vi "Destroy.vi"(8 "Error In":errorcluster, 11 "reference in":refnum<class "DinnerMenuEnum.lvclass">) -> (0 "Error Out":errorcluster, 3 "reference out":refnum<class "DinnerMenuEnum.lvclass">)   [LabVIEW 2020, in "DinnerMenuEnum.lvclass"]
uses:
  DinnerMenuEnum.lvclass
  DinnerMenuEnum.lvclass/DinnerMenuEnum.ctl
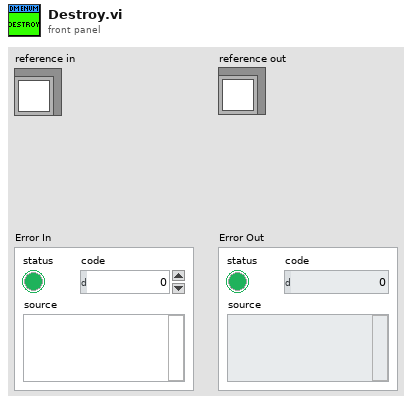
[diagram p1: front panel]
types:
  T1 = typedef "DinnerMenuEnum.lvclass/ObjectAttributes.ctl" = cluster{"_items":refnum<class "Menu.lvclass">[], "_position":i32, "IEnumerator.Current":refnum<class>, "Current":refnum<class "Menu.lvclass">}
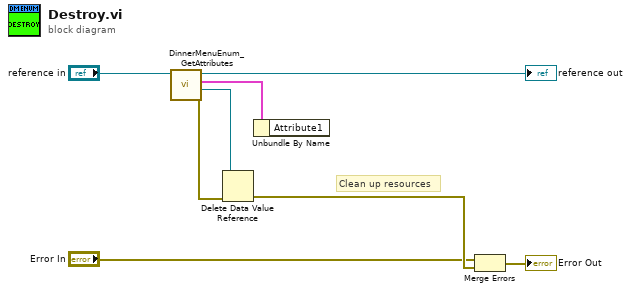
[diagram p0: block diagram]
diagram:
  # "Clean up resources"
  n1 = call "DinnerMenuEnum_GetAttributes.vi"("reference in"="reference in") -> ("error out"=w5:errorcluster, "DataRef"=w4:refnum<data-value>, "Data"=w3:T1, "reference out"=→"reference out":refnum<class "DinnerMenuEnum.lvclass">)  [unwired: 7 in]
  n2 = Delete Data Value Reference(data value reference=w4, error in=w5) -> (error out=w2:errorcluster)  [unwired: 1 out]
  n3 = Unbundle By Name(w3) -> ()  [unwired: 1 out]
  n4 = Merge Errors("Error In", w2) -> (→"Error Out":errorcluster)
